vi "_Create (Protected).vi"(8 "error in (no error)":errorcluster, 11 "BufferedArray in":refnum<class "BufferedArray.lvclass">) -> (0 "error out":errorcluster, 3 "BufferedArray out":refnum<class "BufferedArray.lvclass">)   [LabVIEW 2013, in "LapDog.Collections.v1.Lists.Implementations.lvlib" / "BufferedArray.lvclass"]
doc: "This method is invoked when the List:Create method is called. Child implementations should override this method to initialize or obtain any runtime resource needed. \n\nChild classes do not need to wrap the code in an error case."
uses:
  BufferedArray.lvclass
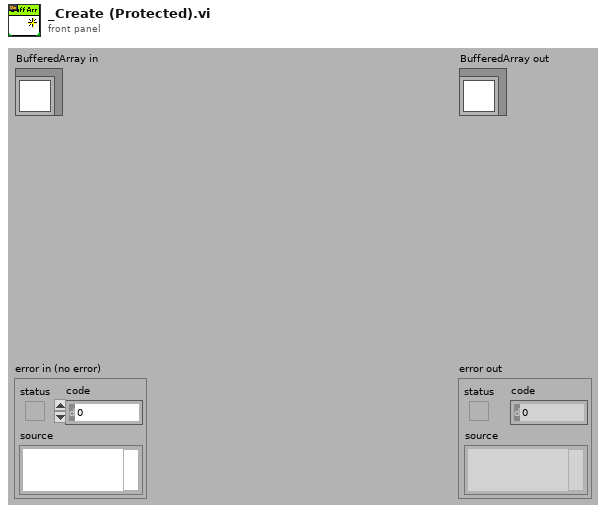
[diagram p1: front panel]
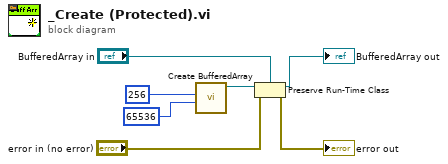
[diagram p0: block diagram]
diagram:
  n1 = call "Create BufferedArray.vi"("Maximum Buffer Increment (65536)"=65536, "Minimum Buffer Size (256)"=256 ("Minimum Buffer Increment (256)")) -> ("BufferedArray out"=w7:refnum<class "BufferedArray.lvclass">)  [unwired: 8 in, 1 out]
  n2 = Preserve Run-Time Class(object in=w7, error in="error in (no error)", 2:"BufferedArray in") -> (object out=→"BufferedArray out":refnum<class "BufferedArray.lvclass">, error out=→"error out":errorcluster)
